vi "MV3D RGBD Map Depth To Point Cloud.vi"(9 "pstPointCloudImage":T1, 10 "pstDepthImage":T1, 11 "handle":u32) -> (1 "pstPointCloudImage out":T1, 2 "pstDepthImage out":T1, 3 "handle out":u32, 5 "function return":i32)   [LabVIEW 2015, in "Mv3dRgbd.lvlib"]
doc: "MV3D_RGBD_API MV3D_RGBD_STATUS MV3D_RGBD_MapDepthToPointCloud(void* handle, MV3D_RGBD_IMAGE_DATA* pstDepthImage, MV3D_RGBD_IMAGE_DATA* pstPointCloudImage);"
uses:
  <userlib>/Mv3dRgbd/Mv3dRgbd.lvlib
  <userlib>/Mv3dRgbd/Mv3dRgbd.dll
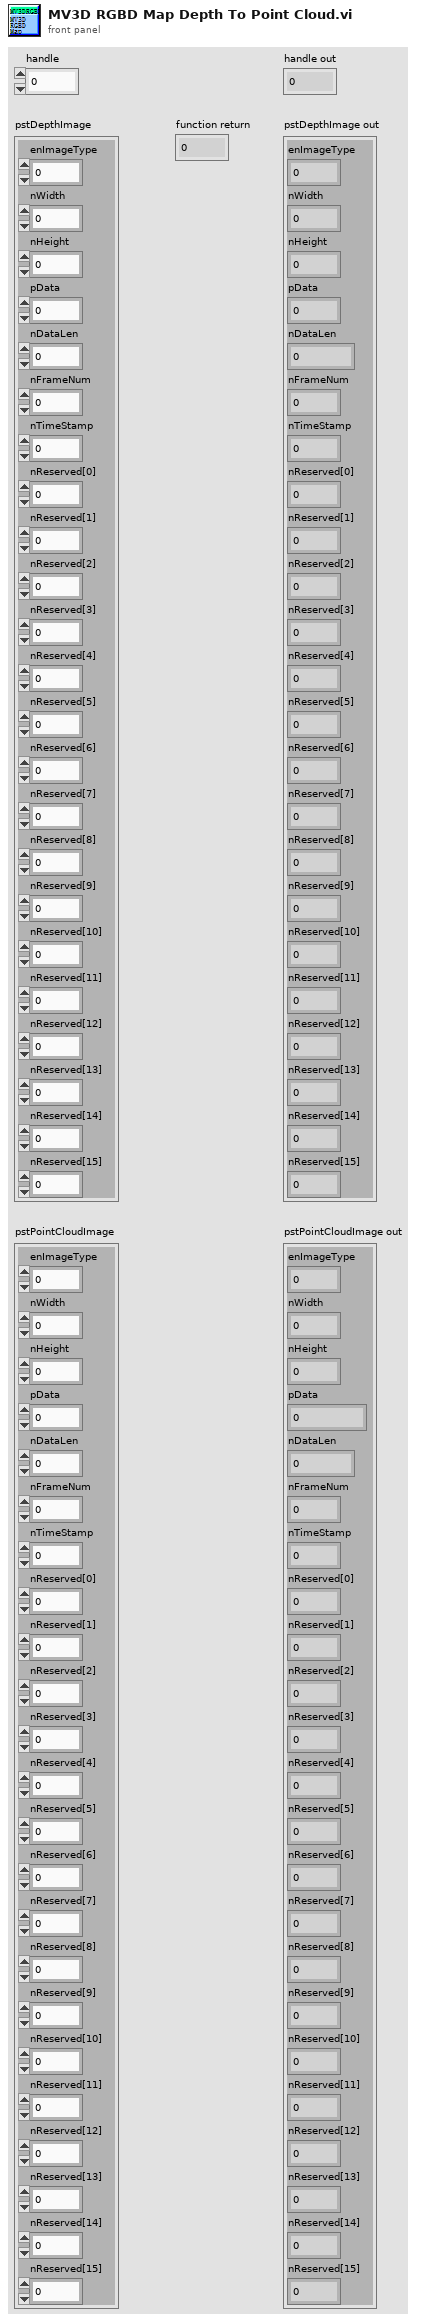
[diagram p1: front panel]
types:
  T1 = cluster{"enImageType":i32, "nWidth":u32, "nHeight":u32, "pData":u32, "nDataLen":u32, "nFrameNum":u32, "nTimeStamp":i64, "nReserved[0]":u8, "nReserved[1]":u8, "nReserved[2]":u8, "nReserved[3]":u8, "nReserved[4]":u8, "nReserved[5]":u8, "nReserved[6]":u8, "nReserved[7]":u8, "nReserved[8]":u8, "nReserved[9]":u8, "nReserved[10]":u8, "nReserved[11]":u8, "nReserved[12]":u8, "nReserved[13]":u8, "nReserved[14]":u8, "nReserved[15]":u8}
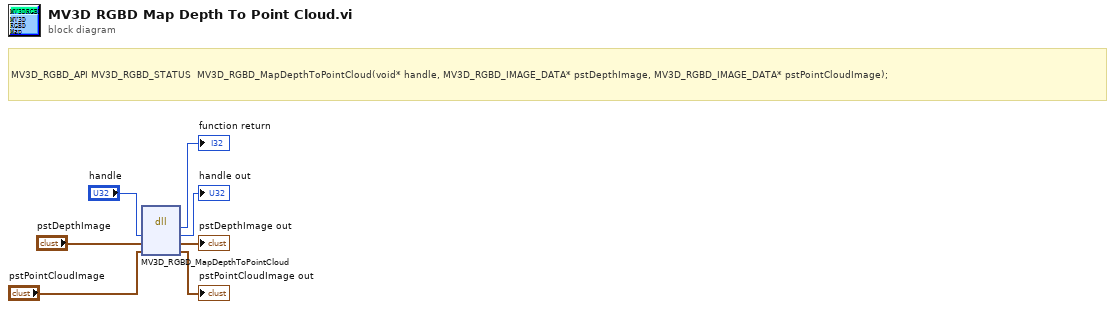
[diagram p0: block diagram]
diagram:
  # "MV3D_RGBD_API MV3D_RGBD_STATUS  MV3D_RGBD_MapDepthToPointCloud(void* handle, MV3D_RGBD_IMAGE_DATA* pstDepthImage, MV3D_RGBD_IMAGE_DATA* pstPointCloudImage);"
  n1 = dll-call lib="C:/Program Files (x86)/National Instruments/LabVIEW 2015/user.lib/Mv3dRgbd/Mv3dRgbd.*" fn="MV3D_RGBD_MapDepthToPointCloud"("handle"="handle", "pstDepthImage"="pstDepthImage", "pstPointCloudImage"="pstPointCloudImage") -> ("返回类型"=→"function return":i32, "handle"=→"handle out":u32, "pstDepthImage"=→"pstDepthImage out":T1, "pstPointCloudImage"=→"pstPointCloudImage out":T1)  [unwired: 3 in, 2 out]
